vi "Write Single Coil.vi"(6 "timeout ms (1000)":i32=1000, 8 "error in (no error)":errorcluster, 9 "Value":bool, 10 "Address":u16, 11 "TCP Network Connection in":refnum<k5>) -> (0 "error out":errorcluster, 3 "TCP Network Connection out":refnum<k5>)   [LabVIEW 2023, in "Modbus TCP Micro.lvlib"]
uses:
  Modbus TCP Micro.lvlib
  Modbus Functions.ctl
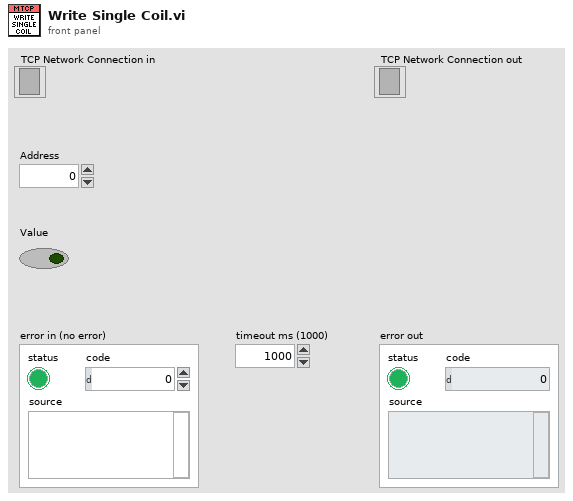
[diagram p1: front panel]
types:
  T1 = typedef "Modbus TCP Micro.lvlib/Modbus Functions.ctl" = u8
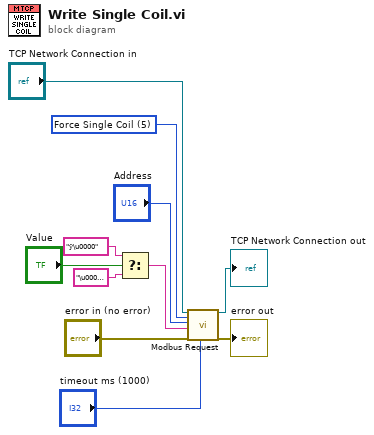
[diagram p0: block diagram]
diagram:
  w1 = T1 5 items=["None"=0, "Read Coil Status"=1, "Read Input Status"=2, "Read Holding Registers"=3, "Read Input Registers"=4, "Force Single Coil"=5, "Preset Single Register"=6, "Force Multiple Coils"=15, "Preset Multiple Registers"=16] ("Function Codes")
  n1 = Select(t="ÿ\u0000" ("data string"), s="Value", f="\u0000\u0000" ("data string")) -> (s? t:f=w8:string)
  n2 = call "Modbus Request.vi"("TCP Network Connection in"="TCP Network Connection in", "Function Codes"=w1, "Start Address"="Address", "Payload"=w8, "error in (no error)"="error in (no error)", "timeout ms (1000)"="timeout ms (1000)") -> ("TCP Network Connection out"=→"TCP Network Connection out":refnum<k5>, "error out"=→"error out":errorcluster)  [unwired: 8 in, 4 out]
